vi "SwissSPAD Live_FGPA Clock Base.vi"(8 "error in (no error)":errorcluster) -> (0 "error out":errorcluster, 3 "Clock Base":dbl[unit])   [LabVIEW 2021]
uses:
  SwissSPAD Live_Settings List.ctl
  Variant/Variant to Data/Variant to Data.lvlib
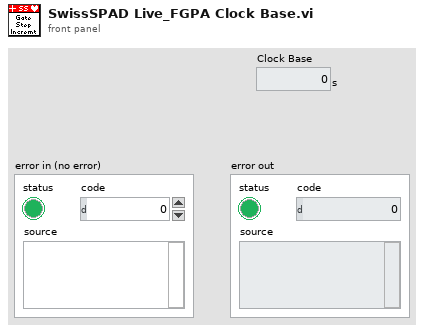
[diagram p1: front panel]
types:
  T1 = typedef "SwissSPAD Live_Settings List.ctl" = enum16{"FPGA:Bottom Half", "FPGA:Top Half", "FPGA:Bottom Bitfile Path", "FPGA:Top Bitfile Path", "FPGA:Bottom Bitstream Version", "FPGA:Top Bitstream Version", "FPGA:Auto Reset FPGA", "FPGA:Bottom FPGA Serial Number", "FPGA:Top FPGA Serial Number", "FPGA:Detector PCB Version", "Acquisition Parameters:Microlens", "Acquisition Parameters:SS2 DAQ Parameters", "Acquisition Parameters:Gate Configuration Array", "Acquisition Parameters:SS3 DAQ Parameters", "Acquisition Parameters:Buffer Size (# 8-bit Gates)", "File Information:File Information", "File Information:# Datasets in Series", "File Information:Scrambled File Flag", "File Information:SS3 Gate Slip Correction", "File Information:SS3 Hot Pixel Mismatch Detection", "File Information:Delay between Datasets", "File Information:Save Sum of All Gates Preview", "Image Parameters:Image ROI Information", "Image Parameters:Image Binning Options", "Image Parameters:SS3 Displayed Image", "Image Parameters:Image Display Options", "Image Parameters:Use Histogram Cursors", "Image Parameter:FPGA Data to Display", "UI Settings:Histogram Bins Number", "UI Settings:Use Image Display Options", "UI Settings:Verbose Settings", "UI Settings:Verbose Saving"}
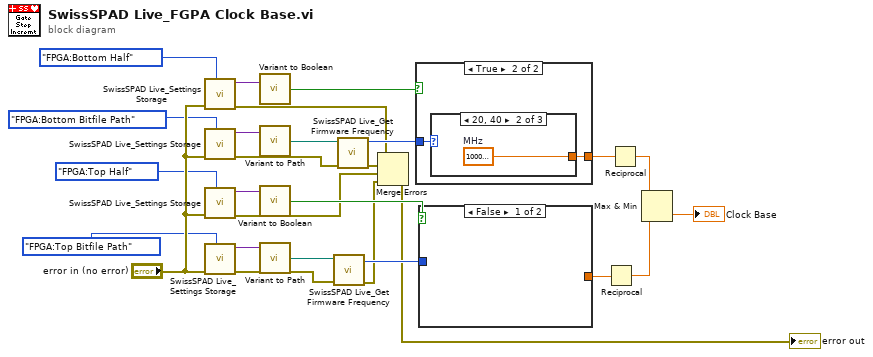
[diagram p0: block diagram]
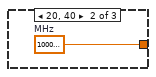
[diagram p3: hidden frame]
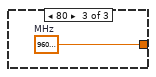
[diagram p4: hidden frame]
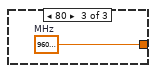
[diagram p7: hidden frame]
diagram:
  n1 = call "SwissSPAD Live_Settings Storage.vi"("Settings List"=SwissSPAD_Live_Settings_List."FPGA:Bottom Half", "Error In"="error in (no error)") -> ("Error Out"=w10:errorcluster, "Variant Data out"=w4:variant)  [unwired: 8 in]
  n2 = call "SwissSPAD Live_Settings Storage.vi"("Settings List"=SwissSPAD_Live_Settings_List."FPGA:Bottom Bitfile Path", "Error In"="error in (no error)") -> ("Error Out"=w24:errorcluster, "Variant Data out"=w3:variant)  [unwired: 8 in]
  n3 = call "SwissSPAD Live_Settings Storage.vi"("Settings List"=SwissSPAD_Live_Settings_List."FPGA:Top Half", "Error In"="error in (no error)") -> ("Error Out"=w12:errorcluster, "Variant Data out"=w2:variant)  [unwired: 8 in]
  n4 = call "SwissSPAD Live_Settings Storage.vi"("Settings List"=SwissSPAD_Live_Settings_List."FPGA:Top Bitfile Path", "Error In"="error in (no error)") -> ("Error Out"=w23:errorcluster, "Variant Data out"=w1:variant)  [unwired: 8 in]
  n5 = call "Variant to Boolean.vi"("Variant"=w4) -> ("Value"=w20:bool)  [unwired: 8 in]
  n6 = call "Variant to Path.vi"("Variant"=w3) -> ("Path"=w26:path)  [unwired: 8 in]
  n7 = call "Variant to Boolean.vi"("Variant"=w2) -> ("Value"=w18:bool)  [unwired: 8 in]
  n8 = call "Variant to Path.vi"("Variant"=w1) -> ("Path"=w25:path)  [unwired: 8 in]
  n9 = call "SwissSPAD Live_Get Firmware Frequency.vi"("Error In"=w23, "Firmware Path"=w25) -> ("Error Out"=w11:errorcluster, "Frequency (MHz)"=w21:i32)  [unwired: 8 in]
  n10 = call "SwissSPAD Live_Get Firmware Frequency.vi"("Error In"=w24, "Firmware Path"=w26) -> ("Error Out"=w13:errorcluster, "Frequency (MHz)"=w22:i32)  [unwired: 8 in]
  n11 = Merge Errors(w10, w13, w12, w11) -> (→"error out":errorcluster)
  n12 = case shown="True" w20 {
    tunnel: w22 -> [_ w29]
    tunnel: [_ w28] -> w19
    frame False {
    }
    frame True {
      n13 = case shown="20, 40" w29 {
        tunnel: [_ w30 w31] -> w28
        frame 0, Default {
        }
        frame 20, 40 {
          w30 = dbl[unit] 1000000000.0  # MHz
        }
        frame 80 {
          w31 = dbl[unit] 960000000.0  # MHz
        }
      }
    }
  }
  n14 = case shown="False" w18 {
    tunnel: w21 -> [_ w33]
    tunnel: [_ w32] -> w17
    frame False {
    }
    frame True {
      n15 = case shown="0, Default" w33 {
        tunnel: [_ w34 w35] -> w32
        frame 0, Default {
        }
        frame 20, 40 {
          w34 = dbl[unit] 1000000000.0  # MHz
        }
        frame 80 {
          w35 = dbl[unit] 960000000.0  # MHz
        }
      }
    }
  }
  n16 = Reciprocal(x=w17) -> (1/x=w15:dbl[unit])
  n17 = Reciprocal(x=w19) -> (1/x=w16:dbl[unit])
  n18 = Max & Min(x=w16, y=w15) -> (min(x,y)=→"Clock Base":dbl[unit])  [unwired: 1 out]
